vi "Take Area Image.vi"(0 "Gantry in":refnum<class "Gantry.lvclass">, 1 "Quality":enum16{"perfect", "high", "medium", "low"}(ring), 5 "Image Center":refnum<class "Vec3d.lvclass">, 9 "Field of View":cluster{"Size-X(mm)":dbl, "Size-Y(mm)":dbl}, 11 "error in (no error)":errorcluster, 12 "Image Name":string="composite image", 13 "Slider Reference":refnum<vi>, 14 "Interrupt Reference":refnum<vi>) -> (4 "Gantry out":refnum<class "Gantry.lvclass">, 6 "Physical Image":T1, 15 "error out":errorcluster)   [LabVIEW 2022 SP3, in "Gantry.lvclass"]
uses:
  Gantry.lvclass
  Utils/Type Definitions/Physical Image.ctl
  Vec3d Class/Vec3d.lvclass
  <vilib>/vision/Image Controls.llb/IMAQ Image.ctl
  FlexWorktable/FlexWorktable.lvclass
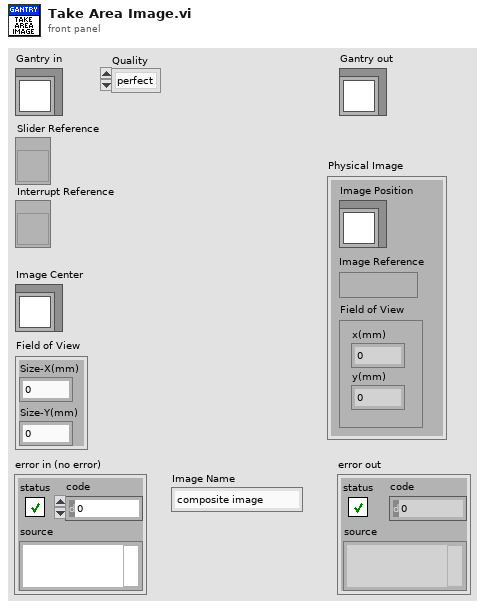
[diagram p1: front panel]
types:
  T1 = typedef "Physical Image.ctl" = cluster{"Image Position":refnum<class "Vec3d.lvclass">, "Image Reference":T2, "Field of View":cluster{"x(mm)":dbl, "y(mm)":dbl}}
  T2 = typedef "IMAQ Image.ctl" = refnum<image>
  T3 = typedef "FlexWorktable.lvclass/Camera State.ctl" = cluster{"Group":i32, "Open?":bool, "Driver":T4, "serial number":string, "Field of View":cluster{"x-mm":dbl, "y-mm":dbl}, "Rotation":T5, "Vertical Mirror":bool}
  T4 = typedef "Vision.lvlib/camera driver.ctl" = enum16{"none", "ueye"}
  T5 = typedef "Camera Rotation.ctl" = enum16{"0", "90", "180", "270"}
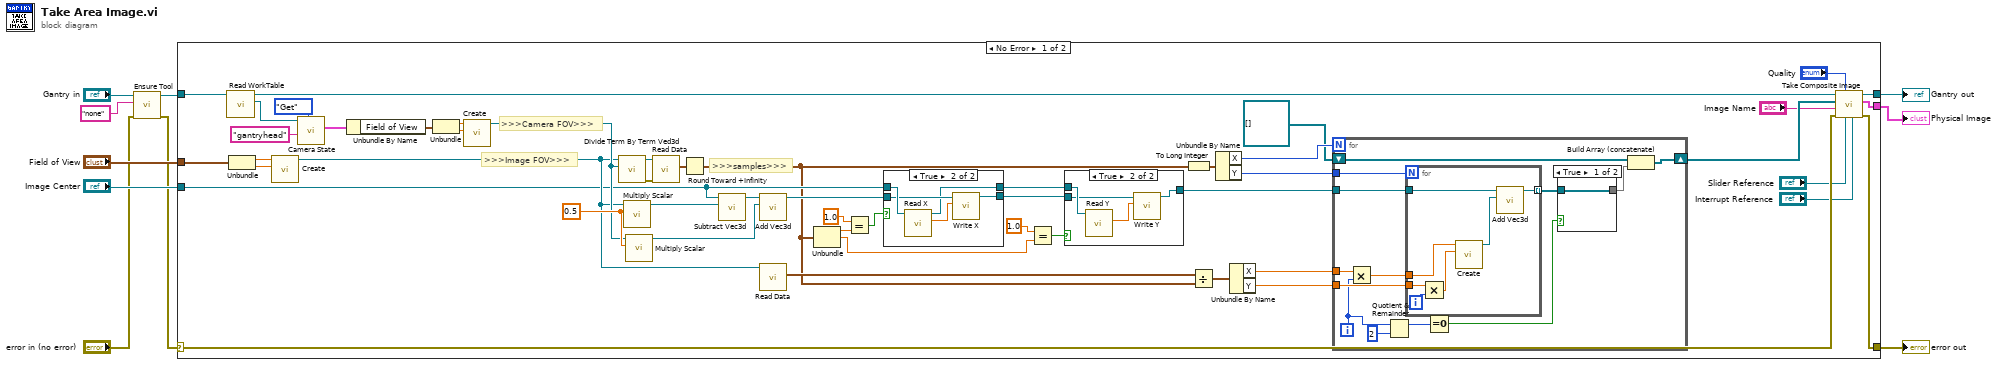
[diagram p0: block diagram]
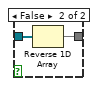
[diagram p4: hidden frame]
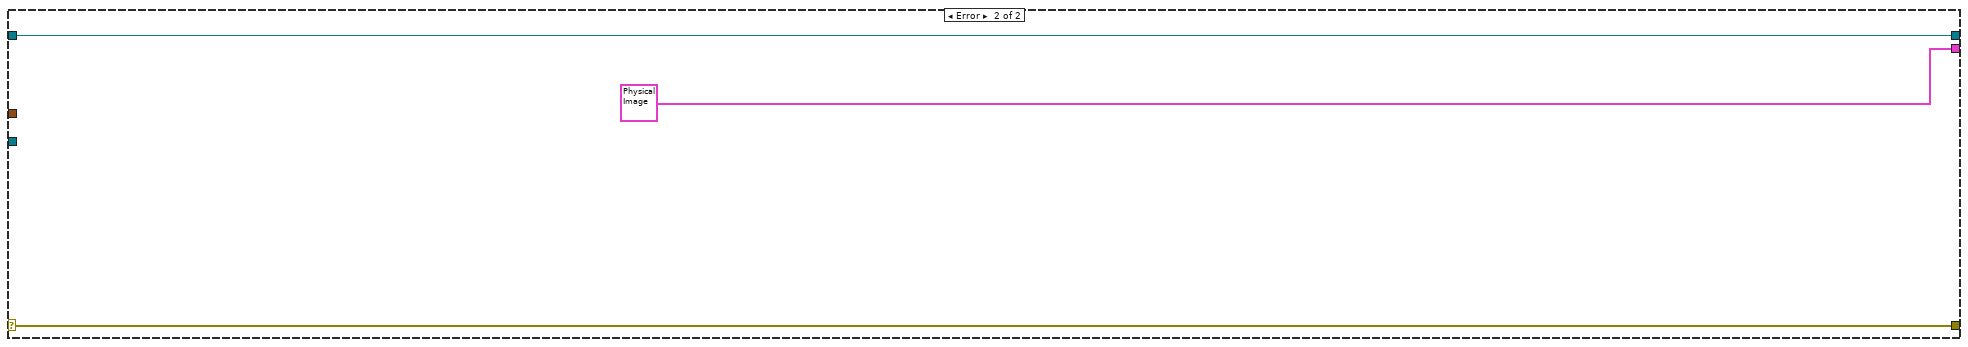
[diagram p5: hidden frame]
diagram:
  n1 = call "Ensure Tool.vi"("error in (no error)"="error in (no error)", "Tool Name"="none", "Gantry in"="Gantry in") -> ("error out"=w2:errorcluster, "Gantry out"=w4:refnum<class "Gantry.lvclass">)  [unwired: 7 in]
  n2 = case shown="No Error" w2 {
    selector: w2 -> [w43 w98]
    tunnel: [w42 w98] -> w8
    tunnel: [w51 w97] -> w7
    tunnel: w4 -> [w15 w97]
    tunnel: "Field of View" -> [w60 _]
    tunnel: "Image Center" -> [w30 _]
    tunnel: [w41 T1 {"Image Position"=refnum, "Image Reference"=refnum, "Field of View"={"x(mm)"=0.0, "y(mm)"=0.0}} ("Physical Image")] -> w6
    frame No Error {
      w36 = 0.5 ("Scale")
      # ">>>samples>>>"
      # ">>>Camera FOV>>>"
      # ">>>Image FOV>>>"
      n3 = call-dynamic "Read WorkTable.vi"("Gantry Class in"=w15) -> ("Worktable"=w18:refnum<class "FlexWorktable.lvclass">, "Gantry Class out"=w14:refnum<class "Gantry.lvclass">)  [unwired: 8 in, 1 out]
      n4 = Unbundle(w60) -> ("Size-X(mm)"=w59:dbl, "Size-Y(mm)"=w58:dbl)
      n5 = call "Create.vi"("Y"=w58, "X"=w59) -> ("Vec3d Class out"=w34:refnum<class "Vec3d.lvclass">)  [unwired: 8 in, 1 out]
      n6 = call-dynamic "Camera State.vi"("Get/Set"=enum16{"Get", "Set"}."Get", "Camera Name"="gantryhead", "FlexWorktable in"=w18) -> ("State"=w13:T3)  [unwired: 6 in, 2 out]
      n7 = Unbundle By Name(w13) -> ("Field of View"=w55:cluster{"x-mm":dbl, "y-mm":dbl})
      n8 = Unbundle(w55) -> ("x-mm"=w57:dbl, "y-mm"=w56:dbl)
      n9 = call "Create.vi"("Y"=w56, "X"=w57) -> ("Vec3d Class out"=w35:refnum<class "Vec3d.lvclass">)  [unwired: 8 in, 1 out]
      n10 = call-dynamic "Divide Term By Term Ved3d.vi"("Vec3d in 2"=w35, "Vec3d in 1"=w34) -> ("error out"=w54:errorcluster, "Vec3d Class out"=w53:refnum<class "Vec3d.lvclass">)  [unwired: 8 in]
      n11 = call-dynamic "Multiply Scalar.vi"("Scale"=w36, "Vec3d in"=w34) -> ("Vec3d out"=w37:refnum<class "Vec3d.lvclass">)  [unwired: 8 in, 1 out]
      n12 = call-dynamic "Multiply Scalar.vi"("Scale"=w36, "Vec3d in"=w35) -> ("Vec3d out"=w32:refnum<class "Vec3d.lvclass">)  [unwired: 8 in, 1 out]
      n13 = call-dynamic "Read Data.vi"("error in (no error)"=w54, "Vec3d Class in"=w53) -> ("Data"=w39:cluster{"X":dbl, "Y":dbl, "Z":dbl})  [unwired: 7 in, 2 out]
      n14 = Round Toward +Infinity(x=w39) -> (ceil(x): smallest int >= x=w29:cluster{"X":dbl, "Y":dbl, "Z":dbl})
      n15 = call "Subtract Vec3d.vi"("Vec3d in 2"=w37, "Vec3d in 1"=w30) -> ("Vec3d Class out"=w33:refnum<class "Vec3d.lvclass">)  [unwired: 8 in, 1 out]
      n16 = call-dynamic "Add Vec3d.vi"(10:"Vec3d Class in"=w32, 11:"Vec3d Class in"=w33) -> ("Vec3d Class out"=w31:refnum<class "Vec3d.lvclass">)  [unwired: 8 in, 1 out]
      n17 = call-dynamic "Read Data.vi"("Vec3d Class in"=w34) -> ("Data"=w38:cluster{"X":dbl, "Y":dbl, "Z":dbl})  [unwired: 8 in, 2 out]
      n18 = Unbundle(w29) -> ("X"=w28:dbl, "Y"=w21:dbl)  [unwired: 1 out]
      n19 = Equal?(x=1.0, y=w28) -> (x = y?=w26:bool)
      n20 = case shown="True" w26 {
        tunnel: w31 -> [w66 w71]
        tunnel: w30 -> [w67 w72]
        tunnel: [w67 w69] -> w25
        tunnel: [w66 w68] -> w24
        frame False {
        }
        frame True {
          n21 = call-dynamic "Read X.vi"("Vec3d Class in"=w72) -> ("X"=w70:dbl, "Vec3d Class out"=w69:refnum<class "Vec3d.lvclass">)  [unwired: 8 in, 1 out]
          n22 = call-dynamic "Write X.vi"("X"=w70, "Vec3d Class in"=w71) -> ("Vec3d Class out"=w68:refnum<class "Vec3d.lvclass">)  [unwired: 8 in, 1 out]
        }
      }
      n23 = Equal?(x=1.0, y=w21) -> (x = y?=w20:bool)
      n24 = case shown="True" w20 {
        tunnel: w24 -> [w61 w64]
        tunnel: w25 -> [_ w65]
        tunnel: [w61 w62] -> w23
        frame False {
        }
        frame True {
          n25 = call-dynamic "Read Y.vi"("Vec3d Class in"=w65) -> ("Y"=w63:dbl)  [unwired: 8 in, 2 out]
          n26 = call-dynamic "Write Y.vi"("Y"=w63, "Vec3d Class in"=w64) -> ("Vec3d Class out"=w62:refnum<class "Vec3d.lvclass">)  [unwired: 8 in, 1 out]
        }
      }
      n27 = To Long Integer(number=w29) -> (32bit integer=w49:cluster{"X":i32, "Y":i32, "Z":i32})
      n28 = Divide(x=w38, y=w29) -> (x/y=w52:cluster{"X":dbl, "Y":dbl, "Z":dbl})
      n29 = Unbundle By Name(w49) -> ("X"=w50:i32, "Y"=w48:i32)
      n30 = Unbundle By Name(w52) -> ("X"=w47:dbl, "Y"=w46:dbl)
      n31 = for {
        N: w50 -> [_]
        tunnel: w48 -> [w85]
        tunnel: w47 -> [w84]
        tunnel: w46 -> [w83]
        shift-right: [w80] -> w44
        shift-left: refnum<class "Vec3d.lvclass">[] [] -> [w81]
        tunnel: w23 -> [w79]
        i -> [w78]
        n32 = Multiply(x=w84, y=w78) -> (x*y=w82:dbl)
        n33 = Quotient & Remainder(x=w78, y=2) -> (x-y*floor(x/y)=w76:i32)  [unwired: 1 out]
        n34 = for {
          N: w85 -> [_]
          tunnel: w83 -> [w95]
          tunnel: w82 -> [w92]
          tunnel: [w90] -> w74 mode=indexing
          tunnel: w79 -> [w89]
          i -> [w94]
          n35 = Multiply(x=w95, y=w94) -> (x*y=w93:dbl)
          n36 = call "Create.vi"("Y"=w93, "X"=w92) -> ("Vec3d Class out"=w91:refnum<class "Vec3d.lvclass">)  [unwired: 8 in, 1 out]
          n37 = call-dynamic "Add Vec3d.vi"(10:"Vec3d Class in"=w91, 11:"Vec3d Class in"=w89) -> ("Vec3d Class out"=w90:refnum<class "Vec3d.lvclass">)  [unwired: 8 in, 1 out]
        }
        n38 = Equal To 0?(x=w76) -> (x = 0?=w75:bool)
        n39 = case shown="True" w75 {
          tunnel: w74 -> [w86 w88]
          tunnel: [w86 w87] -> w73
          frame True {
          }
          frame False {
            n40 = Reverse 1D Array(array=w88) -> (reversed array=w87:refnum<class "Vec3d.lvclass">[])
          }
        }
        n41 = Build Array (concatenate)(w81, w73) -> (w80:refnum<class "Vec3d.lvclass">[])
      }
      n42 = call "Take Composite Image.vi"("Interrupt Reference"="Interrupt Reference", "Slider Reference"="Slider Reference", "Quality"="Quality", "error in (no error)"=w43, "Image Name"="Image Name", "Points"=w44, "Gantry in"=w14) -> ("error out"=w42:errorcluster, "Physical Image"=w41:T1, "Gantry out"=w51:refnum<class "Gantry.lvclass">)  [unwired: 2 in]
    }
    frame Error {
    }
  }
  "error out" <- w8
  "Gantry out" <- w7
  "Physical Image" <- w6
